vi "HorstLesen_ECD.vi"(5 "VorwortHorst":string[](array[string]), 6 "Port":i32, 7 "Senden?":bool[](array[boolean]), 8 "Zwischenspeicher":string[](array[string]), 9 "string":string, 10 "SkalierungsfaktorHorst":dbl[](array[numeric])) -> (2 "Zwischenspeicher":string[](array[string]), 3 "Senden?":bool[](array[boolean]))   [LabVIEW 2017]
uses:
  GVMWHorst_ECD.vi
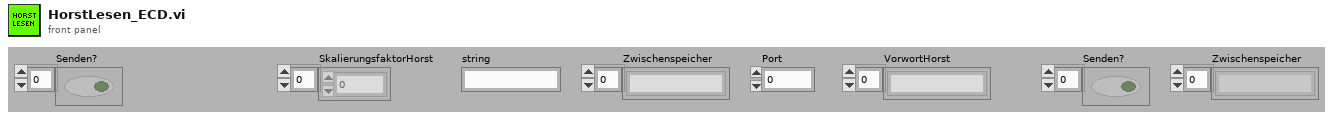
[diagram p1: front panel]
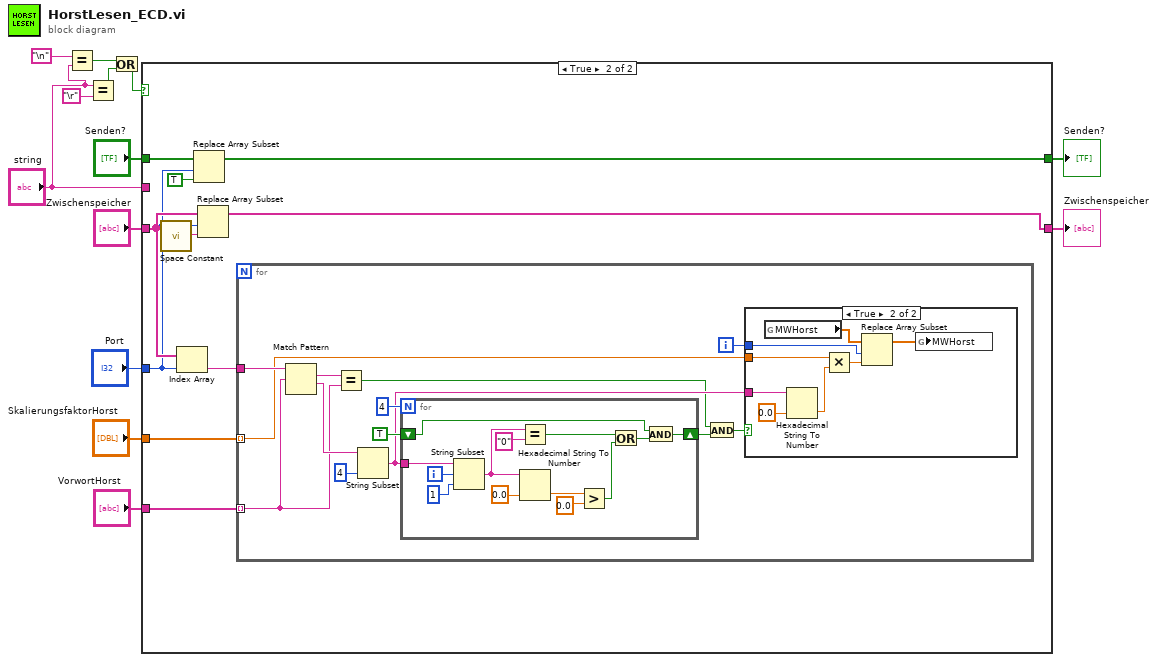
[diagram p0: block diagram]
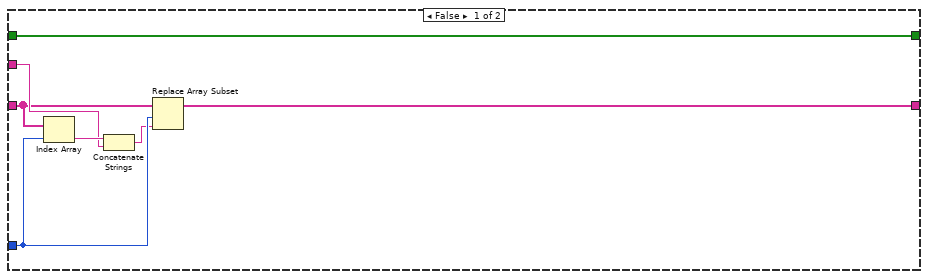
[diagram p2: hidden frame]
diagram:
  n1 = Equal?(x="\n", y="string") -> (x = y?=w3:bool)
  n2 = Equal?(x="string", y="\r") -> (x = y?=w2:bool)
  n3 = Or(x=w3, y=w2) -> (x .or. y?=w1:bool)
  n4 = case shown="True" w1 {
    tunnel: "string" -> [w19 _]
    tunnel: "Zwischenspeicher" -> [w18 w27]
    tunnel: "Port" -> [w17 w26]
    tunnel: [w15 w24] -> w8
    tunnel: "Senden?" -> [w14 w30]
    tunnel: [w14 w28] -> w9
    tunnel: "VorwortHorst" -> [_ w22]
    tunnel: "SkalierungsfaktorHorst" -> [_ w21]
    frame False {
      n5 = Index Array(array=w18, index=w17) -> (element=w20:string)
      n6 = Concatenate Strings(w20, w19) -> (w16:string)
      n7 = Replace Array Subset(array=w18, new element=w16, index=w17) -> (w15:string[])
    }
    frame True {
      n8 = call <vilib>:"Space Constant.vi"() -> ("String"=w25:string)
      n9 = Index Array(array=w27, index=w26) -> (element=w23:string)
      n10 = Replace Array Subset(array=w30, new element=TRUE ("Neues Element/Teil-Array"), index=w26) -> (w28:bool[])
      n11 = Replace Array Subset(array=w27, new element=w25, index=w26) -> (w24:string[])
      n12 = for {
        tunnel: w23 -> [w34]
        tunnel: w22 -> [w32] mode=indexing
        tunnel: w21 -> [w33] mode=indexing
        i -> [w42]
        n13 = Match Pattern(string=w34, regular expression=w32) -> (match substring=w43:string, after substring=w38:string)  [unwired: 1 in, 2 out]
        n14 = Equal?(x=w43, y=w32) -> (x = y?=w36:bool)
        n15 = String Subset(string=w38, length (rest)=4 ("Länge (Rest)")) -> (substring=w37:string)  [unwired: 1 in]
        n16 = for {
          N: 4 -> [_]
          tunnel: w37 -> [w56]
          shift-right: [w44] -> w35
          shift-left: TRUE -> [w45]
          i -> [w55]
          n17 = String Subset(string=w56, offset (0)=w55, length (rest)=1 ("Länge (Rest)")) -> (substring=w51:string)
          n18 = Equal?(x=w51, y="0") -> (x = y?=w52:bool)
          n19 = Hexadecimal String To Number(string=w51, default (0uL)=0.0) -> (number=w49:dbl)  [unwired: 1 in, 1 out]
          n20 = Greater?(x=w49, y=0.0) -> (0:w47:bool)
          n21 = Or(x=w52, y=w47) -> (x .or. y?=w46:bool)
          n22 = And(x=w45, y=w46) -> (x .and. y?=w44:bool)
        }
        n23 = And(x=w36, y=w35) -> (x .and. y?=w31:bool)
        n24 = case shown="True" w31 {
          tunnel: w37 -> [_ w60]
          tunnel: w42 -> [_ w61]
          tunnel: w33 -> [_ w59]
          frame False {
          }
          frame True {
            n25 = global read "GVMWHorst_ECD.vi" "MWHorst"() -> (w58:dbl[])
            n26 = Hexadecimal String To Number(string=w60, default (0uL)=0.0) -> (number=w63:dbl)  [unwired: 1 in, 1 out]
            n27 = Multiply(x=w59, y=w63) -> (x*y=w62:dbl)
            n28 = Replace Array Subset(array=w58, new element=w62, index=w61) -> (w57:dbl[])
            n29 = global write "GVMWHorst_ECD.vi" "MWHorst"(w57) -> ()
          }
        }
      }
    }
  }
  "Senden?" <- w9
  "Zwischenspeicher" <- w8
